vi "Set_IP_Simulation_UE_IP_Address.vi"(8 "error in (no error)":errorcluster, 9 "Cellular Technology":T1="2G", 10 "value":string="10.2.0.1", 11 "Base Station":T2) -> (0 "error out":errorcluster, 3 "Output String":string)   [LabVIEW 2021]
uses:
  Controls/Base_Station_Emulator.ctl
  Controls/Cellular_Technology.ctl
  Controls/TCP_FGV.ctl
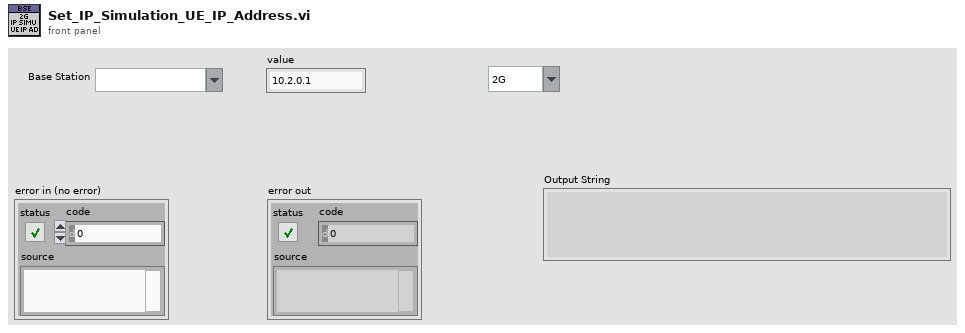
[diagram p1: front panel]
types:
  T1 = typedef "Cellular_Technology.ctl" = string
  T2 = typedef "Base_Station_Emulator.ctl" = string
  T3 = typedef "TCP_FGV.ctl" = enum16{"Open", "Read", "Write", "Close"}
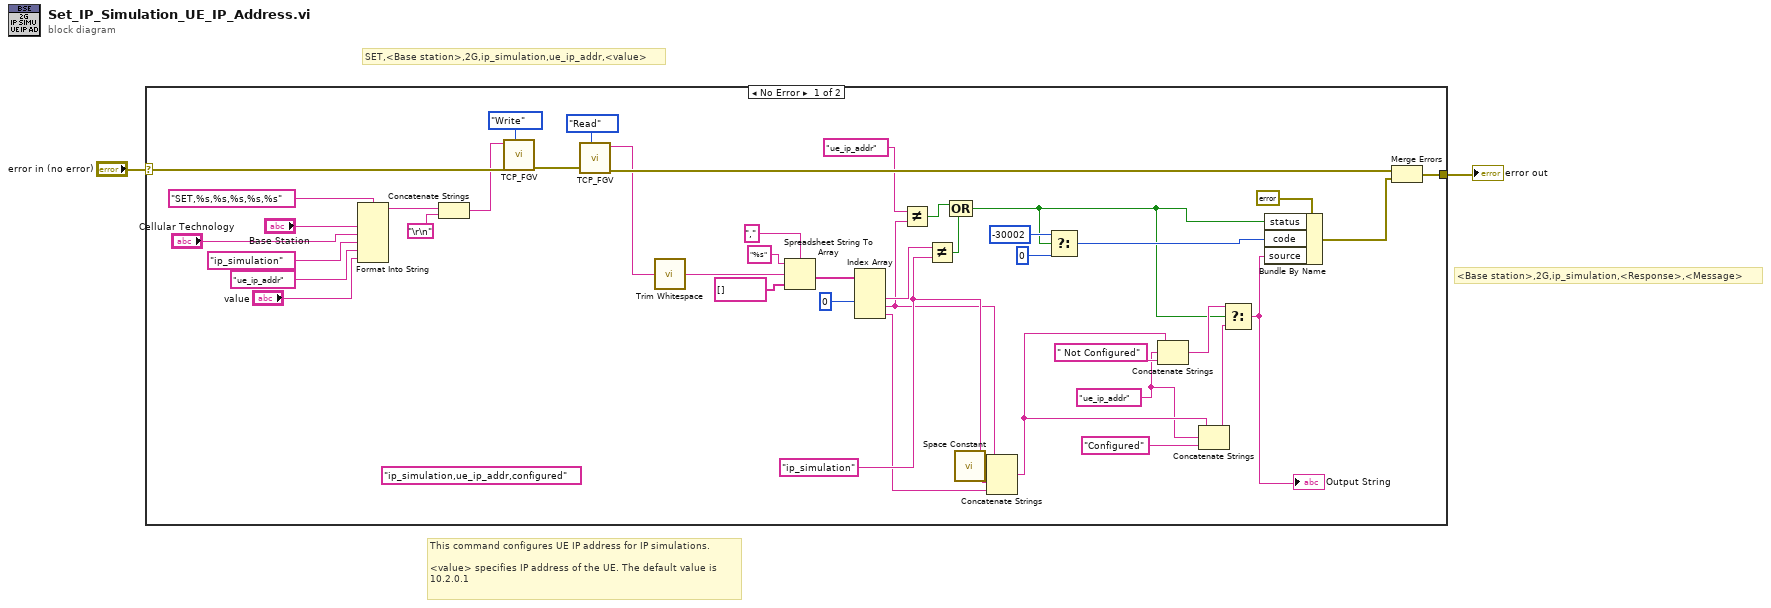
[diagram p0: block diagram]
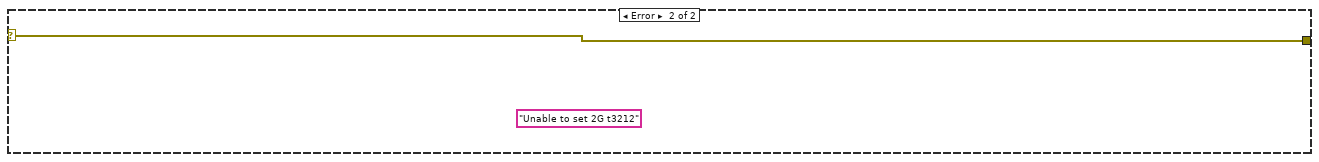
[diagram p2: hidden frame]
diagram:
  # "<Base station>,2G,ip_simulation,<Response>,<Message>"
  # "This command configures UE IP address for IP simulations.\n \n<value> specifies IP address of the UE. The default value is \n10.2.0.1"
  # "SET,<Base station>,2G,ip_simulation,ue_ip_addr,<value>"
  n1 = case shown="No Error" "error in (no error)" {
    selector: "error in (no error)" -> [w42 w46]
    tunnel: [w26 w46] -> w1
    frame No Error {
      w3 = "ue_ip_addr"
      (unwired) "ip_simulation,ue_ip_addr,configured" ("format string")
      w19 = "ip_simulation" ("format string")
      n2 = Format Into String(format string="SET,%s,%s,%s,%s,%s", "Base Station", "Cellular Technology", "ip_simulation", "ue_ip_addr", "value") -> (resulting string=w22:string)  [unwired: 2 in, 1 out]
      n3 = Concatenate Strings(w22, "\r\n") -> (w21:string)
      n4 = call "TCP_FGV.vi"("Command"=w21, "error in (no error)"=w42, "Operation"=TCP_FGV."Write") -> ("error out"=w27:errorcluster)  [unwired: 6 in, 1 out]
      n5 = call "TCP_FGV.vi"("error in (no error)"=w27, "Operation"=TCP_FGV."Read") -> ("Data Out"=w16:string, "error out"=w29:errorcluster)  [unwired: 7 in]
      n6 = call <vilib>:"Trim Whitespace.vi"("string"=w16) -> ("trimmed string"=w40:string)  [unwired: 1 in]
      n7 = Spreadsheet String To Array(delimiter (Tab)=",", format string="%s", spreadsheet string=w40, array type (2D Dbl)=string[] []) -> (array=w37:string[])
      n8 = Index Array(array=w37, index #2=0 ("index")) -> (element #2=w30:string, element #3=w12:string, element #4=w17:string)  [unwired: 3 in, 1 out]
      n9 = Not Equal?(x="ue_ip_addr", y=w12) -> (x != y?=w38:bool)
      n10 = Not Equal?(x=w30, y=w19) -> (x != y?=w39:bool)
      n11 = Compound Arithmetic op=OR(w38, w39) -> (w5:bool)
      n12 = call <vilib>:"Space Constant.vi"() -> ("String"=w18:string)
      n13 = Concatenate Strings(w19, w18, w12, w18, w17) -> (w6:string)
      n14 = Select(t=-30002 ("code"), s=w5, f=0 ("code")) -> (s? t:f=w41:i32)
      n15 = Concatenate Strings(w6, w3, " Not Configured" ("string")) -> (w8:string)
      n16 = Concatenate Strings(w6, w3, "Configured" ("string")) -> (w9:string)
      n17 = Select(t=w8, s=w5, f=w9) -> (s? t:f=w4:string)
      "Output String" <- w4
      n18 = Bundle By Name(cluster=errorcluster {"status"=FALSE, "code"=0, "source"=""} ("error constant"), "status"=w5, "code"=w41, "source"=w4) -> (w28:errorcluster)
      n19 = Merge Errors(w29, w28) -> (w26:errorcluster)
    }
    frame Error {
      (unwired) "Unable to set 2G t3212" ("source")
    }
  }
  "error out" <- w1
